vi "CANBootloader.vi"() -> ()   [LabVIEW 2010]
uses:
  <vilib>/Utility/miscctls.llb/LVRowAndColumnTypeDef.ctl
  usb2can/USB2XXX.dll
panel:
  out "NodeAddr":i32
  out "pVersion out":u32
  in  "pVersion":u32
  in  "pType":u32
  out "Node Position":T1
  in  "pInitConfig":T2
  in  "pCmdList":T3
  in  "Device Index":i32(ring) items=["0", "1", "2", "3", "4", "5"]
  out "固件更新进度":i32(slide) scale=0.0..4284.0
  in  "Upgrate":bool
  out "NodeNum":u16
  in  "扫描节点":bool
  out "扫描进度":u16(slide) max=9 scale=0.0..299.0
  in  "EndAddr":u16
  in  "StartAddr":u16
  in  "Table Scan Node":string[][](table)
  in  "Table Command":string[][](table)
  in  "stop":bool
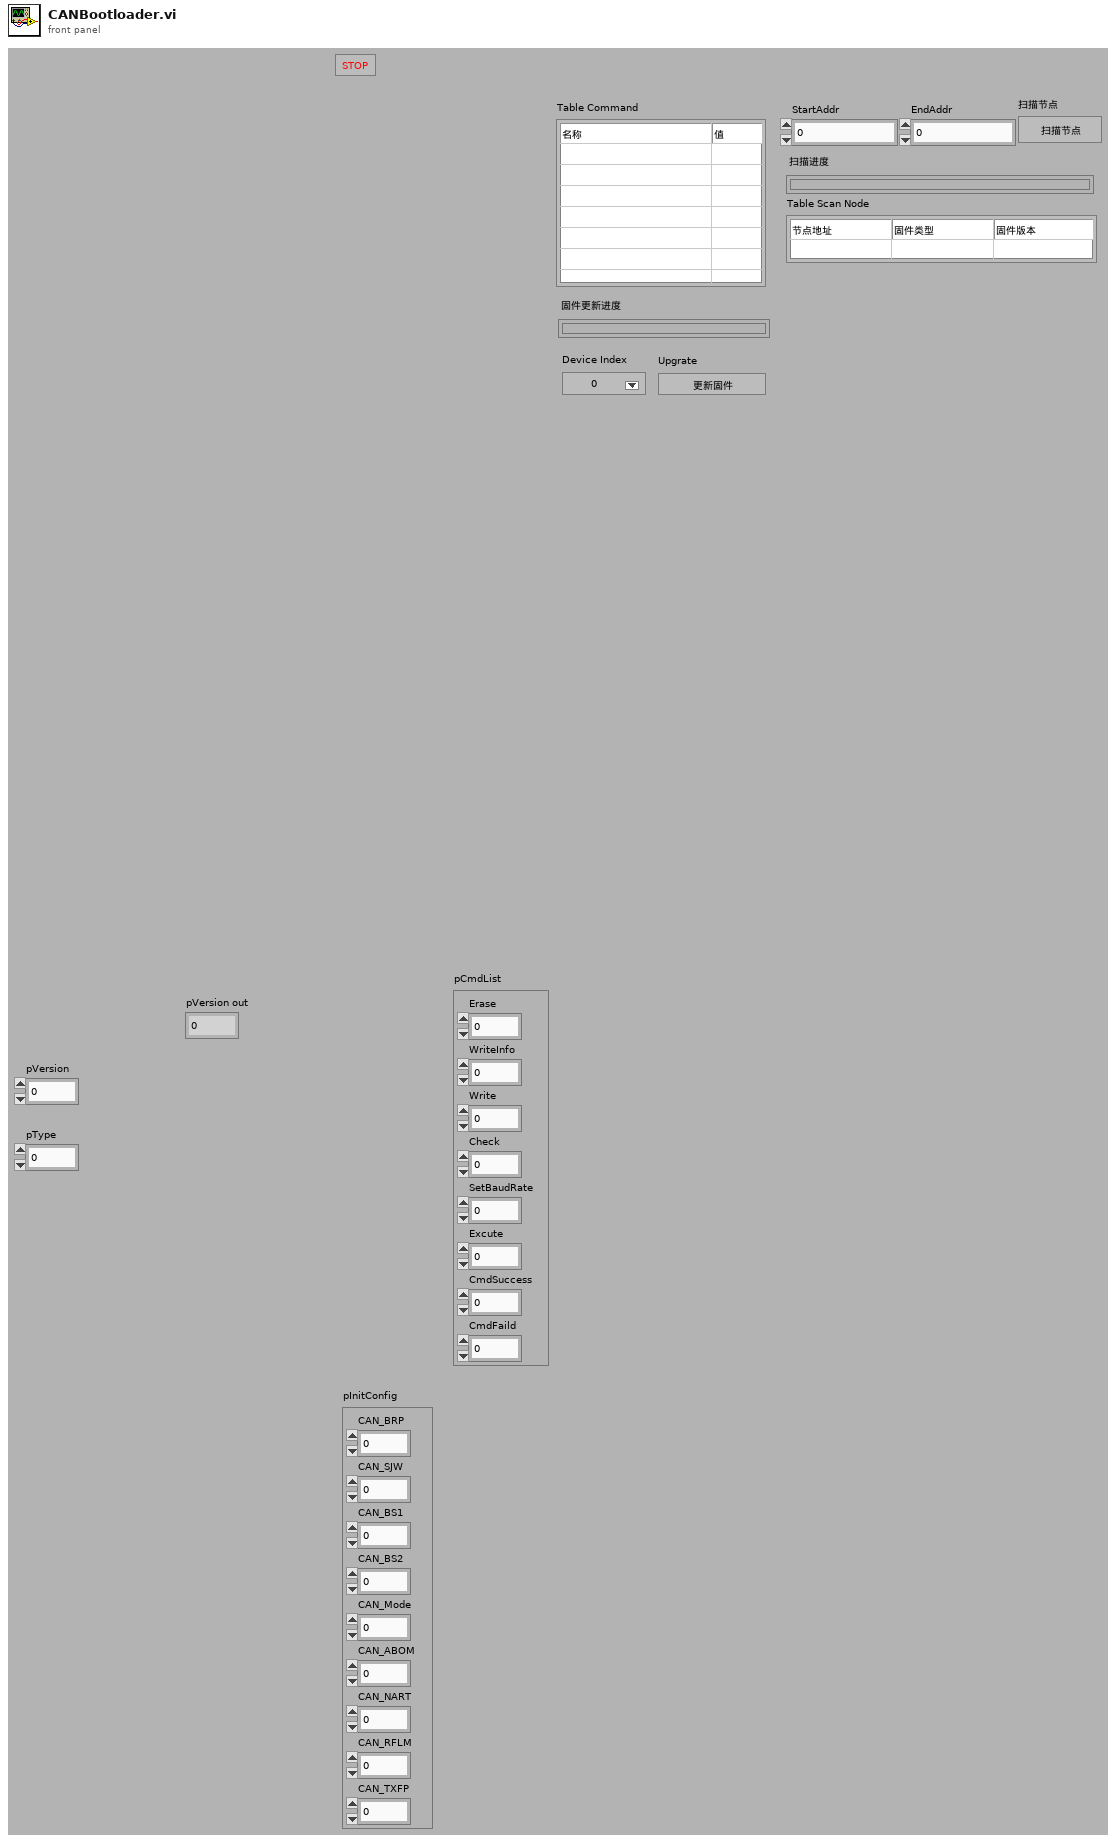
[diagram p1: front panel]
types:
  T1 = typedef "LVRowAndColumnTypeDef.ctl" = cluster{"Row":i32, "Column":i32}
  T2 = cluster{"CAN_BRP":u32, "CAN_SJW":u8, "CAN_BS1":u8, "CAN_BS2":u8, "CAN_Mode":u8, "CAN_ABOM":u8, "CAN_NART":u8, "CAN_RFLM":u8, "CAN_TXFP":u8}
  T3 = cluster{"Erase":u8, "WriteInfo":u8, "Write":u8, "Check":u8, "SetBaudRate":u8, "Excute":u8, "CmdSuccess":u8, "CmdFaild":u8}
  T4 = enum16{"Init", "ScanNode", "Upgrate", "Colse", "Idel"}
  T5 = typedef "LVPoint32TypeDef.ctl" = cluster{"Horizontal":i32, "Vertical":i32}
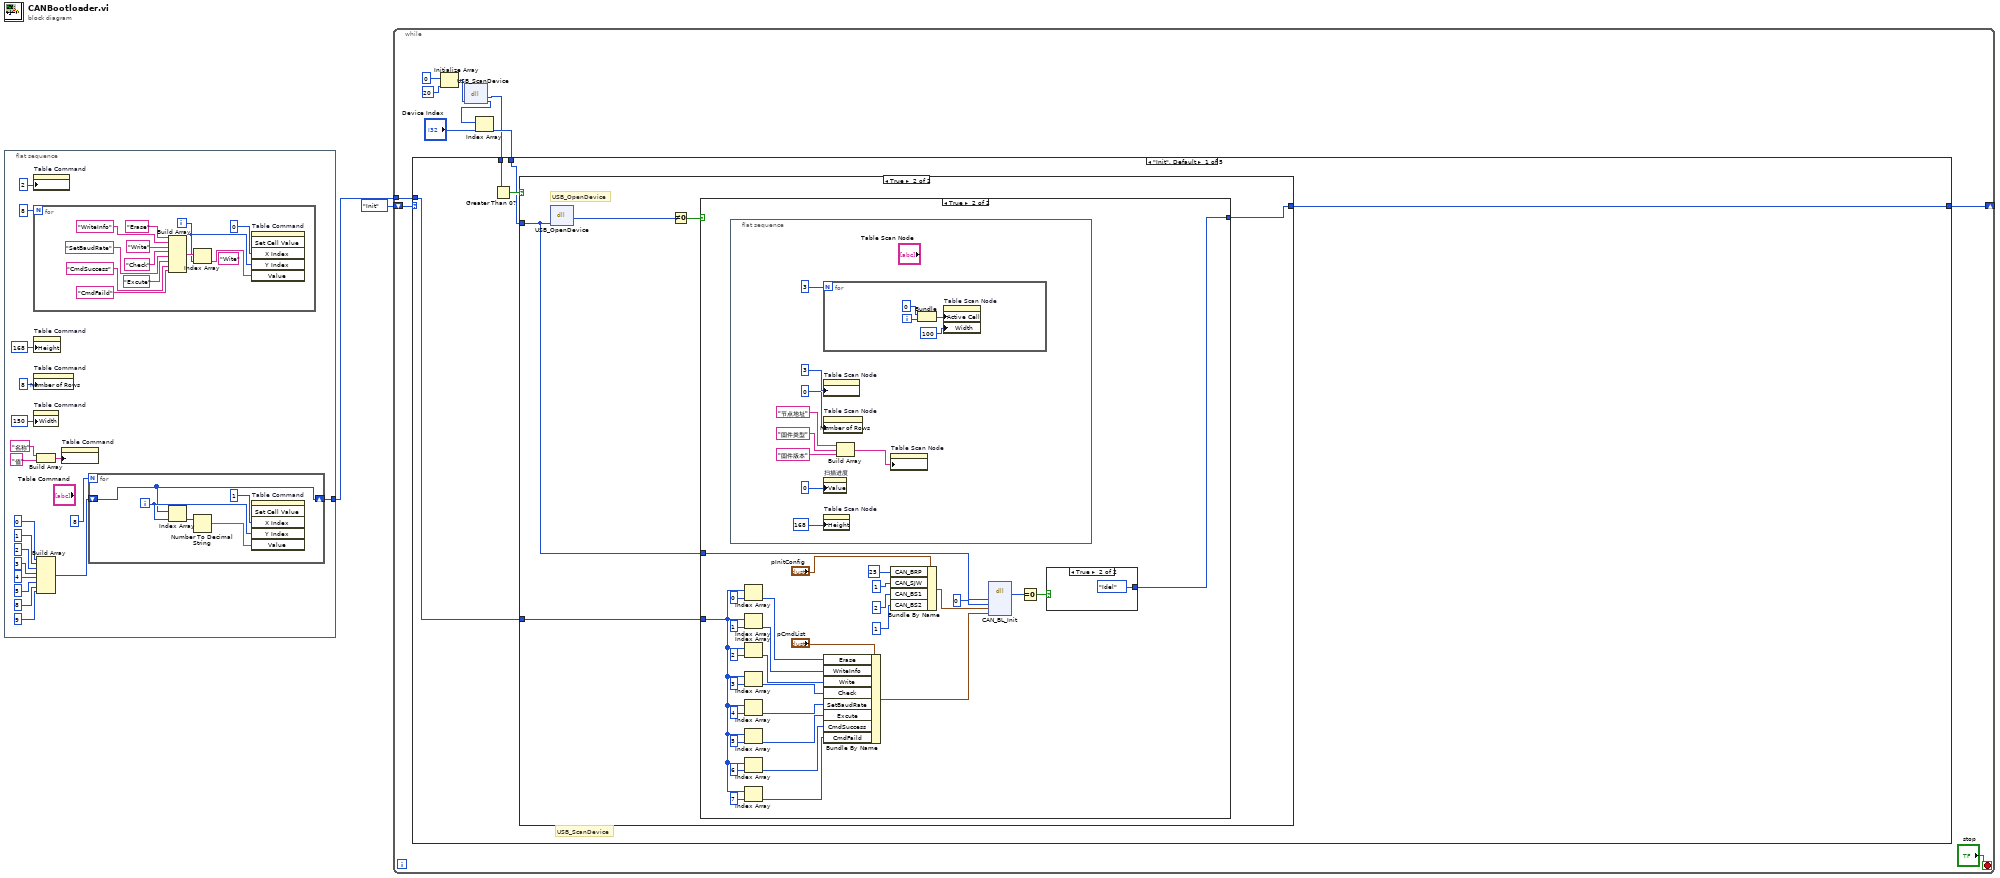
[diagram p0: block diagram]
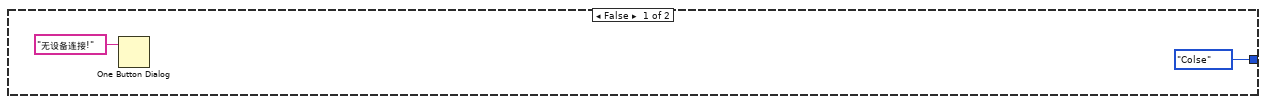
[diagram p2: hidden frame]
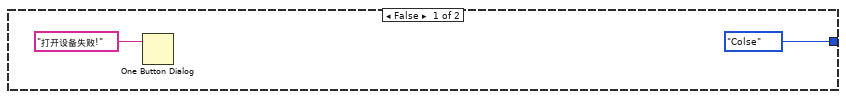
[diagram p3: hidden frame]
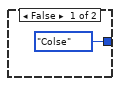
[diagram p4: hidden frame]
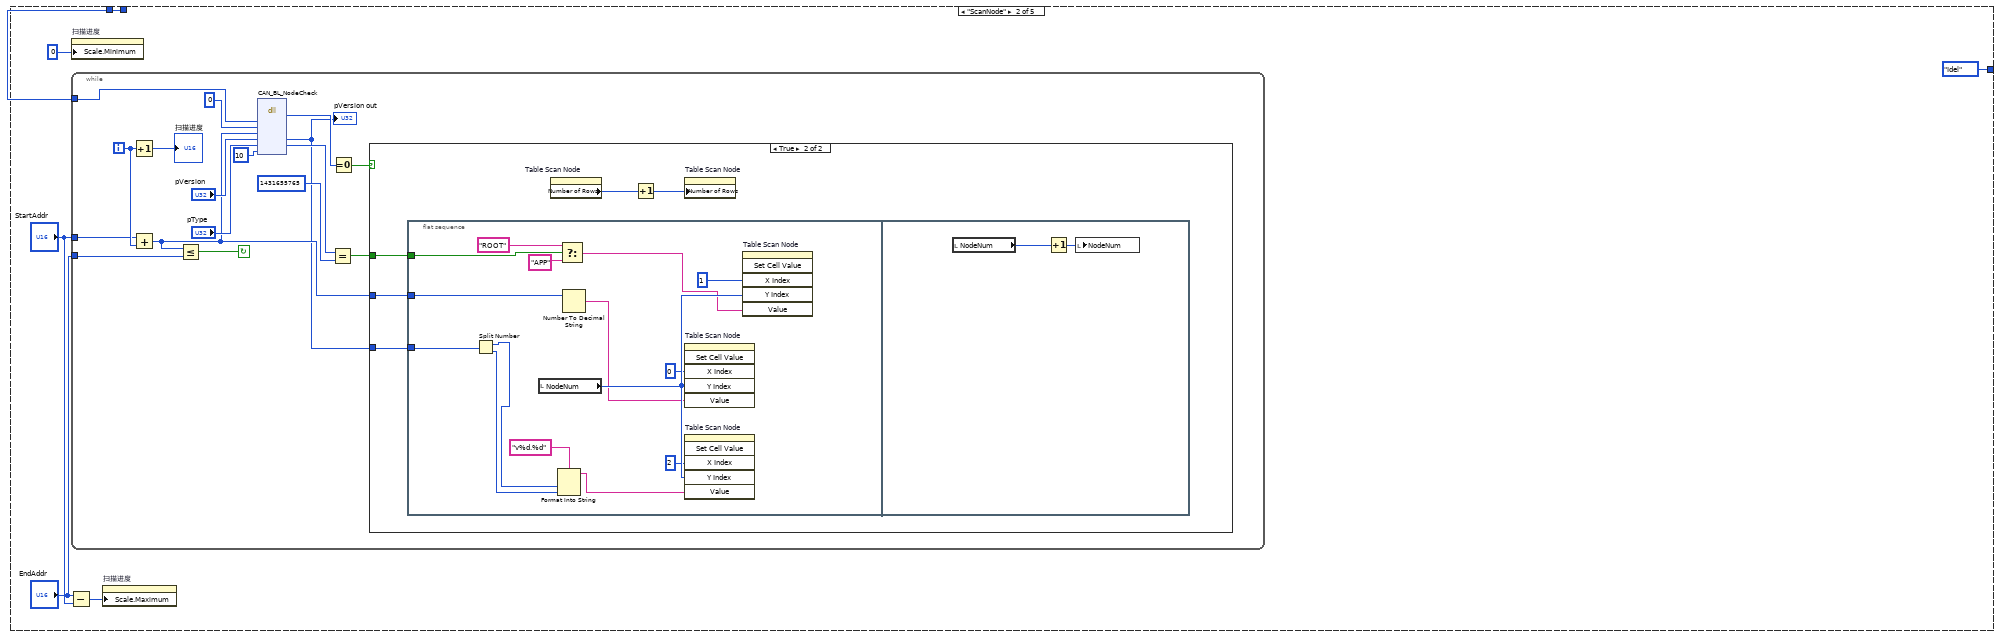
[diagram p5: hidden frame]
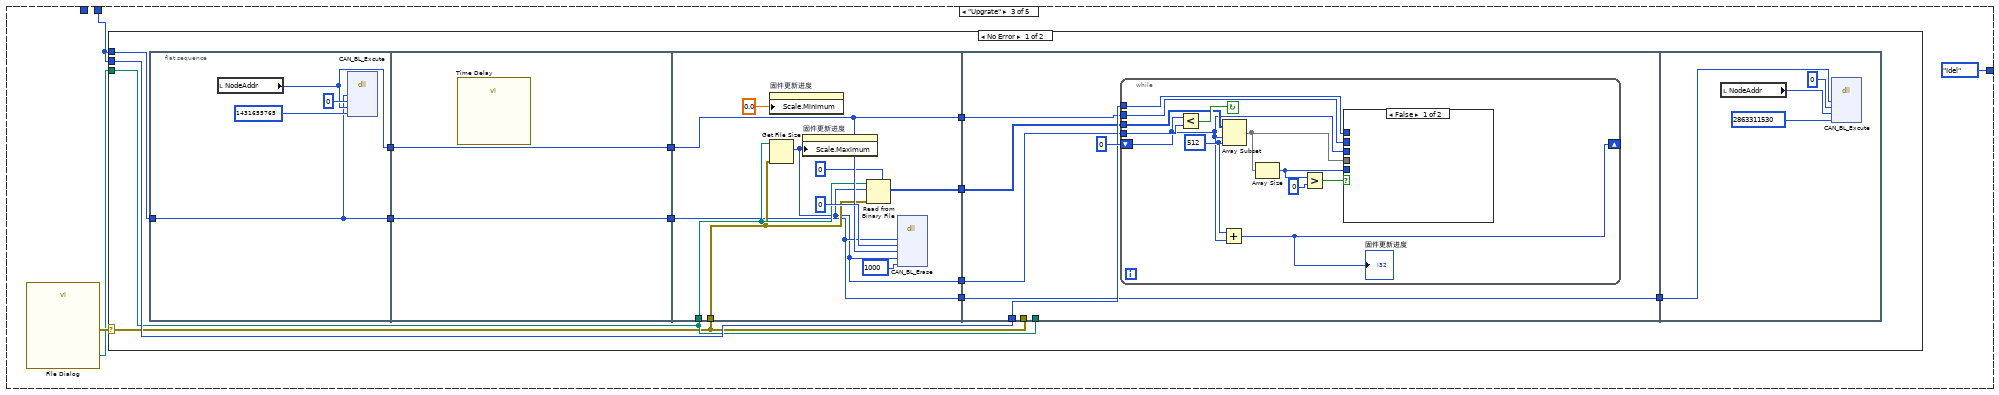
[diagram p7: hidden frame]
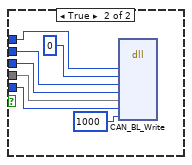
[diagram p8: hidden frame]
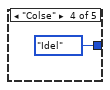
[diagram p10: hidden frame]
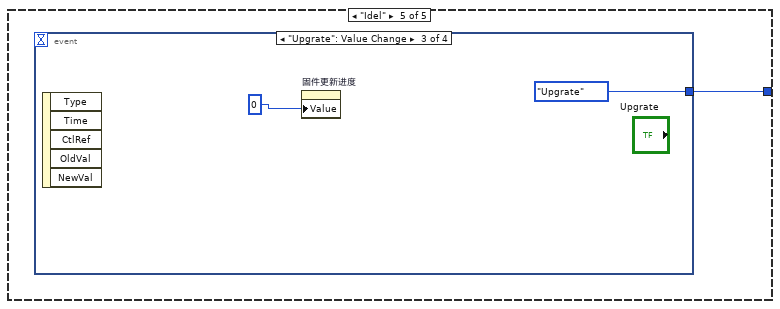
[diagram p11: hidden frame]
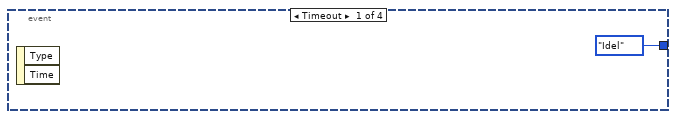
[diagram p12: hidden frame]
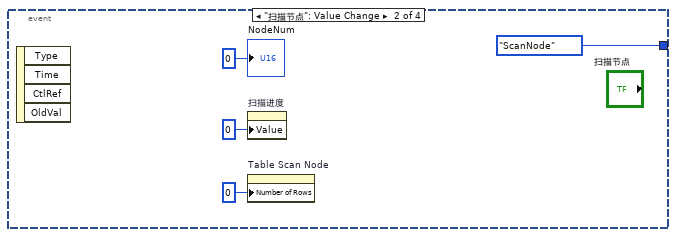
[diagram p13: hidden frame]
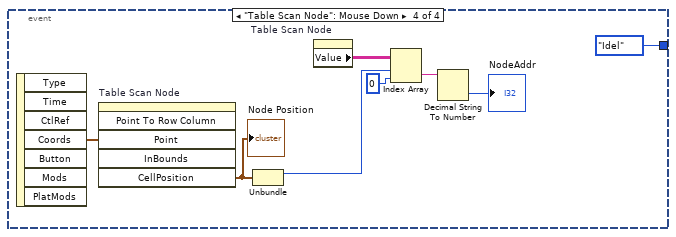
[diagram p14: hidden frame]
diagram:
  n1 = flat-sequence {
    tunnel: [w12] -> w1
    frame #0 {
      n2 = property on="Table Command" class="Tbl (strict)"("Number of Columns"=u32 2) -> ()  [unwired: 2 in, 2 out]
      n3 = for {
        N: 8 -> [_]
        i -> [w28]
        (unwired) "Wite"
        n4 = Build Array("Erase", "WriteInfo", "Write", "Check", "SetBaudRate", "Excute", "CmdSuccess", "CmdFaild") -> (w29:string[])
        n5 = Index Array(array=w29, index=w28) -> (element=w27:string)
        n6 = invoke on="Table Command" class="Tbl (strict)" method="Set Cell Value"("X Index"=u32 0, "Y Index"=w28, "Value"=w27) -> ()  [unwired: 3 in, 6 out]
      }
      n7 = property on="Table Command" class="Tbl (strict)"("Height"=u32 168 ("Size:Height")) -> ()  [unwired: 2 in, 2 out]
      n8 = property on="Table Command" class="Tbl (strict)"("Number of Rows"=u32 8) -> ()  [unwired: 2 in, 2 out]
      n9 = property on="Table Command" class="Tbl (strict)"("Width"=u32 150 ("Active Cell:Cell Size:Width")) -> ()  [unwired: 2 in, 2 out]
      n10 = Build Array("名称", "值") -> (w16:string[])
      n11 = Build Array(u8 0, u8 1, u8 2, u8 3, u8 4, u8 5, u8 8, u8 9) -> (w3:u8[])
      n12 = property on="Table Command" class="Tbl (strict)"("Column Headers[]"=w16) -> ()  [unwired: 2 in, 2 out]
      n13 = for {
        N: 8 -> [_]
        shift-right: [w22] -> w12
        shift-left: w3 -> [w22]
        i -> [w25]
        n14 = Index Array(array=w22, index=w25) -> (element=w24:u8)
        n15 = Number To Decimal String(number=w24) -> (decimal integer string=w23:string)  [unwired: 1 in]
        n16 = invoke on="Table Command" class="Tbl (strict)" method="Set Cell Value"("X Index"=u32 1, "Y Index"=w25, "Value"=w23) -> ()  [unwired: 3 in, 6 out]
      }
    }
  }
  n17 = while {
    shift-right: [w47] -> _
    shift-left: T4."Init" ("Enum") -> [w48]
    tunnel: w1 -> [w46]
    stop <- "stop" stop-if-true
    n18 = Initialize Array(0, 20 ("dimension size")) -> (w43:i32[])
    n19 = dll-call lib="F:/OtherWork/STM32/CAN-Bootloader/software/CANBootloader-Labview/usb2can/USB2XXX.dll" fn="USB_ScanDevice"("pDevNum"=w43) -> ("return type"=w39:i32, "pDevNum"=w44:i32[])  [unwired: 3 in, 2 out]
    n20 = Index Array(array=w44, index="Device Index") -> (element=w40:i32)
    n21 = case shown="\"Init\", Default" w48 {
      tunnel: [w53 T4."Idel" ("Enum") T4."Idel" ("Enum") T4."Idel" ("Enum") w217] -> w47
      tunnel: w40 -> [w51 w111 w154 _ _]
      tunnel: w46 -> [w52 _ _ _ _]
      tunnel: w39 -> [w50 _ _ _ _]
      frame "Init", Default {
        # "USB_ScanDevice"
        n22 = Greater Than 0?(x=w50) -> (x > 0?=w54:bool)
        n23 = case shown="True" w54 {
          tunnel: [T4."Colse" ("Enum") w60] -> w53
          tunnel: w51 -> [_ w58]
          tunnel: w52 -> [_ w59]
          frame False {
            n24 = One Button Dialog(message="无设备连接!") -> ()  [unwired: 1 in, 1 out]
          }
          frame True {
            # "USB_OpenDevice"
            n25 = dll-call lib="F:/OtherWork/STM32/CAN-Bootloader/software/CANBootloader-Labview/usb2can/USB2XXX.dll" fn="USB_OpenDevice"("DevIndex"=w58) -> ("return type"=w61:u8)  [unwired: 4 in, 2 out]
            n26 = Not Equal To 0?(x=w61) -> (x != 0?=w57:bool)
            n27 = case shown="True" w57 {
              tunnel: [T4."Colse" ("Enum") w64] -> w60
              tunnel: w59 -> [_ w71]
              tunnel: w58 -> [_ w67]
              frame False {
                n28 = One Button Dialog(message="打开设备失败!") -> ()  [unwired: 1 in, 1 out]
              }
              frame True {
                n29 = flat-sequence {
                  frame #0 {
                    n30 = for {
                      N: 3 -> [_]
                      i -> [w108]
                      n31 = Bundle("Number of Rows"=u32 0, w108) -> (w106:cluster{"Number of Rows":u32, i32})  [unwired: 1 in]
                      n32 = property on="Table Scan Node" class="Tbl (strict)"("Active Cell"=w106, "Width"=u32 100 ("Active Cell:Cell Size:Width")) -> ()  [unwired: 2 in, 2 out]
                    }
                    n33 = property on="Table Scan Node" class="Tbl (strict)"("Number of Columns"=u32 3) -> ()  [unwired: 2 in, 2 out]
                    n34 = property on="Table Scan Node" class="Tbl (strict)"("Number of Rows"=u32 0) -> ()  [unwired: 2 in, 2 out]
                    n35 = property on="扫描进度" class="Slide (strict)"("Value"=u16 0 ("扫描进度")) -> ()  [unwired: 2 in, 2 out]
                    n36 = property on="Table Scan Node" class="Tbl (strict)"("Height"=u32 168 ("Size:Height")) -> ()  [unwired: 2 in, 2 out]
                    n37 = Build Array("节点地址", "固件类型", "固件版本") -> (w102:string[])
                    n38 = property on="Table Scan Node" class="Tbl (strict)"("Column Headers[]"=w102) -> ()  [unwired: 2 in, 2 out]
                  }
                }
                n39 = Index Array(array=w71, index=0) -> (element=w86:u8)
                n40 = Index Array(array=w71, index=1) -> (element=w78:u8)
                n41 = Index Array(array=w71, index=2) -> (element=w77:u8)
                n42 = Index Array(array=w71, index=3) -> (element=w76:u8)
                n43 = Index Array(array=w71, index=4) -> (element=w75:u8)
                n44 = Index Array(array=w71, index=5) -> (element=w74:u8)
                n45 = Index Array(array=w71, index=6) -> (element=w73:u8)
                n46 = Index Array(array=w71, index=7) -> (element=w72:u8)
                n47 = Bundle By Name(cluster="pCmdList", "Erase"=w86, "WriteInfo"=w78, "Write"=w77, "Check"=w76, "SetBaudRate"=w75, "Excute"=w74, "CmdSuccess"=w73, "CmdFaild"=w72) -> (w69:T3)
                n48 = Bundle By Name(cluster="pInitConfig", "CAN_BRP"=u32 25, "CAN_SJW"=u8 1, "CAN_BS1"=u8 2, "CAN_BS2"=u8 1) -> (w70:T2)
                n49 = dll-call lib="F:/OtherWork/STM32/CAN-Bootloader/software/CANBootloader-Labview/usb2can/USB2XXX.dll" fn="CAN_BL_Init"("DevIndex"=w67, "CANIndex"=0, "pInitConfig"=w70, "pCmdList"=w69) -> ("return type"=w66:i32)  [unwired: 7 in, 2 out]
                n50 = Equal To 0?(x=w66) -> (x = 0?=w65:bool)
                n51 = case shown="True" w65 {
                  tunnel: [T4."Colse" ("Enum") T4."Idel" ("Enum")] -> w64
                  frame False {
                  }
                  frame True {
                  }
                }
              }
            }
          }
        }
      }
      frame "ScanNode" {
        n52 = Subtract(x="EndAddr", y="StartAddr") -> (x-y=w113:u16)
        n53 = property on="扫描进度" class="Slide (strict)"("Scale.Minimum"=u8 0 ("Response to Value Outside Limits:Minimum")) -> ()  [unwired: 2 in, 2 out]
        n54 = while {
          tunnel: w111 -> [w127]
          tunnel: "StartAddr" -> [w121]
          tunnel: "EndAddr" -> [w120]
          i -> [w123]
          stop <- w122 continue-if-true
          n55 = Increment(x=w123) -> (x+1=→"扫描进度":i32)
          n56 = Add(x=w121, y=w123) -> (x+y=w119:i32)
          n57 = Less Or Equal?(x=w119, y=w120) -> (x <= y?=w122:bool)
          n58 = dll-call lib="F:/OtherWork/STM32/CAN-Bootloader/software/CANBootloader-Labview/usb2can/USB2XXX.dll" fn="CAN_BL_NodeCheck"("DevIndex"=w127, "CANIndex"=0, "NodeAddr"=w119, "pVersion"="pVersion", "pType"="pType", "TimeOut"=u32 10) -> ("return type"=w126:i32, "pVersion"=w115:u32, "pType"=w118:u32)  [unwired: 7 in, 2 out]
          "pVersion out" <- w115
          n59 = Equal?(x=w118, y=u32 1431655765) -> (x = y?=w116:bool)
          n60 = Equal To 0?(x=w126) -> (x = 0?=w124:bool)
          n61 = case shown="True" w124 {
            tunnel: w119 -> [_ w136]
            tunnel: w116 -> [_ w133]
            tunnel: w115 -> [_ w132]
            frame False {
            }
            frame True {
              n62 = flat-sequence {
                tunnel: w136 -> [w146]
                tunnel: w133 -> [w143]
                tunnel: w132 -> [w141]
                frame #0 {
                  n63 = Split Number(x=w141) -> (hi(x)=w139:u16, lo(x)=w138:u16)
                  n64 = local read "NodeNum"() -> (w151:u16)
                  n65 = Format Into String(format string="v%d.%d", w139, w138) -> (resulting string=w137:string)  [unwired: 2 in, 1 out]
                  n66 = Select(t="ROOT" ("Value"), s=w143, f="APP" ("Value")) -> (s? t:f=w142:string)
                  n67 = Number To Decimal String(number=w146) -> (decimal integer string=w150:string)  [unwired: 1 in]
                  n68 = invoke on="Table Scan Node" class="Tbl (strict)" method="Set Cell Value"("X Index"=u32 0, "Y Index"=w151, "Value"=w150) -> ()  [unwired: 3 in, 6 out]
                  n69 = invoke on="Table Scan Node" class="Tbl (strict)" method="Set Cell Value"("X Index"=u32 2, "Y Index"=w151, "Value"=w137) -> ()  [unwired: 3 in, 6 out]
                  n70 = invoke on="Table Scan Node" class="Tbl (strict)" method="Set Cell Value"("X Index"=u32 1, "Y Index"=w151, "Value"=w142) -> ()  [unwired: 3 in, 6 out]
                }
                frame #1 {
                  n71 = local read "NodeNum"() -> (w153:u16)
                  n72 = Increment(x=w153) -> (x+1=w152:u16)
                  n73 = local write "NodeNum"(w152) -> ()
                }
              }
              n74 = property on="Table Scan Node" class="Tbl (strict)"() -> ("Number of Rows"=w134:u32)  [unwired: 2 in, 2 out]
              n75 = Increment(x=w134) -> (x+1=w135:u32)
              n76 = property on="Table Scan Node" class="Tbl (strict)"("Number of Rows"=w135) -> ()  [unwired: 2 in, 2 out]
            }
          }
        }
        n77 = property on="扫描进度" class="Slide (strict)"("Scale.Maximum"=w113) -> ()  [unwired: 2 in, 2 out]
      }
      frame "Upgrate" {
        n78 = call "File Dialog"() -> ("selected path"=w155:path, "error out"=w156:errorcluster)  [unwired: 12 in, 2 out]
        n79 = case shown="No Error" w156 {
          selector: w156 -> [w162 _]
          tunnel: w155 -> [w163 _]
          tunnel: w154 -> [w170 _]
          tunnel: w154 -> [w169 _]
          frame No Error {
            n80 = flat-sequence {
              tunnel: w170 -> [w171]
              tunnel: [w172] -> w168
              tunnel: [w171] -> w165
              tunnel: w168 -> [w176]
              tunnel: [w176] -> w167
              tunnel: w165 -> [w175]
              tunnel: [w175] -> w164
              tunnel: w167 -> [w185]
              tunnel: [w185] -> w166
              tunnel: w164 -> [w178]
              tunnel: w163 -> [w183]
              tunnel: w162 -> [w182]
              tunnel: [w180] -> w161
              tunnel: [w177] -> w160
              tunnel: [w178] -> w158
              tunnel: w163 -> [_]
              tunnel: w162 -> [_]
              tunnel: w169 -> [w191]
              tunnel: w166 -> [w190]
              tunnel: w161 -> [w189]
              tunnel: w160 -> [w188]
              tunnel: [w187] -> w159
              tunnel: w158 -> [w187]
              tunnel: w159 -> [w213]
              frame #0 {
                n81 = local read "NodeAddr"() -> (w172:i32)
                n82 = dll-call lib="F:/OtherWork/STM32/CAN-Bootloader/software/CANBootloader-Labview/usb2can/USB2XXX.*" fn="CAN_BL_Excute"("DevIndex"=w171, "CANIndex"=0, "NodeAddr"=w172, "Type"=u32 1431655765) -> ()  [unwired: 8 in, 2 out]
              }
              frame #1 {
                n83 = call "Time Delay"() -> ()  [unwired: 11 in, 1 out]
              }
              frame #2 {
                n84 = property on="固件更新进度" class="Slide (strict)"("Scale.Minimum"=0.0 ("Scale.Range:Minimum")) -> ()  [unwired: 2 in, 2 out]
                n85 = Get File Size(file=w183, error in=w182) -> (size (in bytes)=w177:i64)  [unwired: 2 out]
                n86 = property on="固件更新进度" class="Slide (strict)"("Scale.Maximum"=w177) -> ()  [unwired: 2 in, 2 out]
                n87 = Read from Binary File(5:u8 0, 8:w182, 10:w177, 11:w183) -> (2:w180:u8[])  [unwired: 2 in, 3 out]
                n88 = dll-call lib="F:/OtherWork/STM32/CAN-Bootloader/software/CANBootloader-Labview/usb2can/USB2XXX.*" fn="CAN_BL_Erase"("DevIndex"=w178, "CANIndex"=0, "NodeAddr"=w185, "FlashSize"=w177, "TimeOut"=u32 1000) -> ()  [unwired: 9 in, 2 out]
              }
              frame #3 {
                n89 = while {
                  shift-right: [w193] -> _
                  shift-left: 0 -> [w194]
                  tunnel: w188 -> [w203]
                  tunnel: w189 -> [w202]
                  tunnel: w191 -> [w197]
                  tunnel: w190 -> [w196]
                  stop <- w204 continue-if-true
                  w201 = 512 ("length")
                  n90 = Less?(x=w194, y=w203) -> (x < y?=w204:bool)
                  n91 = Add(x=w201, y=w194) -> (x+y=w193:i32)
                  "固件更新进度" <- w193
                  n92 = Array Subset(array=w202, index=w194, length=w201) -> (w195:u8[])
                  n93 = Array Size(array=w195) -> (size(s)=w198:i32)
                  n94 = Greater?(x=w198, y=0) -> (0:w199:bool)
                  n95 = case shown="False" w199 {
                    tunnel: w198 -> [_ w206]
                    tunnel: w197 -> [_ w211]
                    tunnel: w196 -> [_ w209]
                    tunnel: w194 -> [_ w208]
                    tunnel: w195 -> [_ w207]
                    frame False {
                    }
                    frame True {
                      n96 = dll-call lib="F:/OtherWork/STM32/CAN-Bootloader/software/CANBootloader-Labview/usb2can/USB2XXX.*" fn="CAN_BL_Write"("DevIndex"=w211, "CANIndex"=0, "NodeAddr"=w209, "AddrOffset"=w208, "pData"=w207, "DataNum"=w206, "TimeOut"=u32 1000) -> ()  [unwired: 11 in, 2 out]
                    }
                  }
                }
              }
              frame #4 {
                n97 = local read "NodeAddr"() -> (w212:i32)
                n98 = dll-call lib="F:/OtherWork/STM32/CAN-Bootloader/software/CANBootloader-Labview/usb2can/USB2XXX.*" fn="CAN_BL_Excute"("DevIndex"=w213, "CANIndex"=0, "NodeAddr"=w212, "Type"=u32 2863311530) -> ()  [unwired: 8 in, 2 out]
              }
            }
          }
          frame Error {
          }
        }
      }
      frame "Colse" {
      }
      frame "Idel" {
        n99 = event shown="[2] \"Upgrate\": Value Change" {
          selector: _ -> [_ _ _ _]
          dyn-events: _ -> [_ _ _ _]
          timeout: _ -> [_ _ _ _]
          tunnel: [T4."Idel" ("Enum") T4."ScanNode" ("Enum") T4."Upgrate" ("Enum") T4."Idel" ("Enum")] -> w217
          event Timeout {
            n100 = event-data() -> ()  [unwired: 1 in, 2 out]
          }
          event "扫描节点": Value Change {
            n101 = event-data() -> ()  [unwired: 1 in, 4 out]
            n102 = property on="扫描进度" class="Slide (strict)"("Value"=u16 0 ("扫描进度")) -> ()  [unwired: 2 in, 2 out]
            n103 = property on="Table Scan Node" class="Tbl (strict)"("Number of Rows"=u32 0) -> ()  [unwired: 2 in, 2 out]
            "NodeNum" <- u16 0 ("NodeNum")
          }
          event "Upgrate": Value Change {
            n104 = event-data() -> ()  [unwired: 1 in, 5 out]
            n105 = property on="固件更新进度" class="Slide (strict)"("Value"=u8 0 ("固件更新进度")) -> ()  [unwired: 2 in, 2 out]
          }
          event "Table Scan Node": Mouse Down {
            n106 = event-data() -> ("Coords"=w232:T5)  [unwired: 1 in, 6 out]
            n107 = invoke on="Table Scan Node" class="Tbl (strict)" method="Point To Row Column"("Point"=w232) -> ("CellPosition"=w229:T1)  [unwired: 5 in, 5 out]
            "Node Position" <- w229
            n108 = Unbundle(w229) -> ("Row"=w228:i32)  [unwired: 1 out]
            n109 = property on="Table Scan Node" class="Tbl (strict)"() -> ("Value"=w230:string[][])  [unwired: 2 in, 2 out]
            n110 = Index Array(array=w230, index (row)=w228, index (col)=0 ("disabled index (col)")) -> (element=w226:string)
            n111 = Decimal String To Number(string=w226) -> (number=→"NodeAddr":i32)  [unwired: 2 in, 1 out]
          }
        }
      }
    }
  }
